vi "Pack string.vi"(8 "error in (no error)":errorcluster, 9 "Argument":variant, 10 "Keyword Name":string, 11 "Python Toolkit in":refnum<class "Python Toolkit.lvclass">) -> (0 "error out":errorcluster, 3 "Python Toolkit out":refnum<class "Python Toolkit.lvclass">)   [LabVIEW 2018, in "Python Toolkit.lvclass"]
doc: "Pass a value to the provided parameter (keyword arg) of a python function"
uses:
  Python Toolkit.lvclass
  Python Toolkit.lvclass/Python Toolkit.ctl
  <vilib>/Enthought/Python Integration Toolkit/Python Integration Toolkit.lvlib
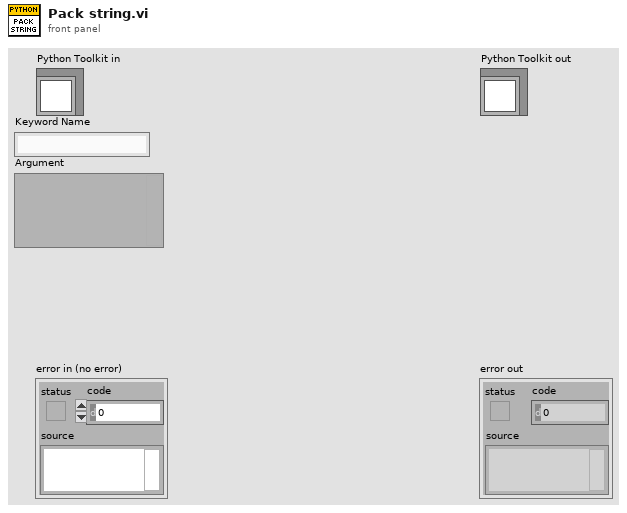
[diagram p1: front panel]
types:
  T1 = typedef "Python Integration Toolkit.lvlib/Session ID.ctl" = u64
  T2 = typedef "Python Integration Toolkit.lvlib/Python Objects.ctl" = variant
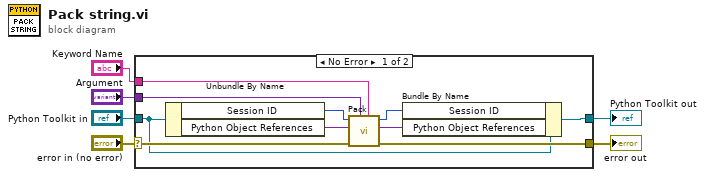
[diagram p0: block diagram]
diagram:
  n1 = case shown="No Error" "error in (no error)" {
    selector: "error in (no error)" -> [w16 w18]
    tunnel: [w15 w18] -> w5
    tunnel: [w12 w17] -> w3
    tunnel: "Python Toolkit in" -> [w13 w17]
    tunnel: "Keyword Name" -> [w9 _]
    tunnel: "Argument" -> [w7 _]
    frame No Error {
      n2 = Unbundle By Name(w13) -> ("Session ID"=w14:T1, "Python Object References"=w8:T2)
      n3 = call <vilib>:"Pack.vi"("Keyword Name"=w9, "Argument"=w7, "error in (no error)"=w16, "Python Object References In"=w8, "Session ID"=w14) -> ("error out"=w15:errorcluster, "Python Object References Out"=w10:T2, "Session ID out"=w11:T1)  [unwired: 4 in]
      n4 = Bundle By Name(cluster=w13, "Session ID"=w11, "Python Object References"=w10) -> (w12:refnum<class "Python Toolkit.lvclass">)
    }
    frame Error {
    }
  }
  "error out" <- w5
  "Python Toolkit out" <- w3
